vi "Peregrine_query_status.vi"(8 "error":errorcluster, 10 "Address":u8, 11 "Handle in":refnum<visa-resource-name>) -> (0 "error out":errorcluster, 1 "Speed":i16, 2 "Position":i32, 3 "Handle out":refnum<visa-resource-name>, 4 "Flags":T1)   [LabVIEW 2019]
panel:
  out "length":i32
  out "unsigned byte array":u8[](array[numeric])
  in  "Flags bundle":T1
  out "Command":i32
  out "Address":u8
  # "Inputs"
  # "Indicators"
  # "Outputs"
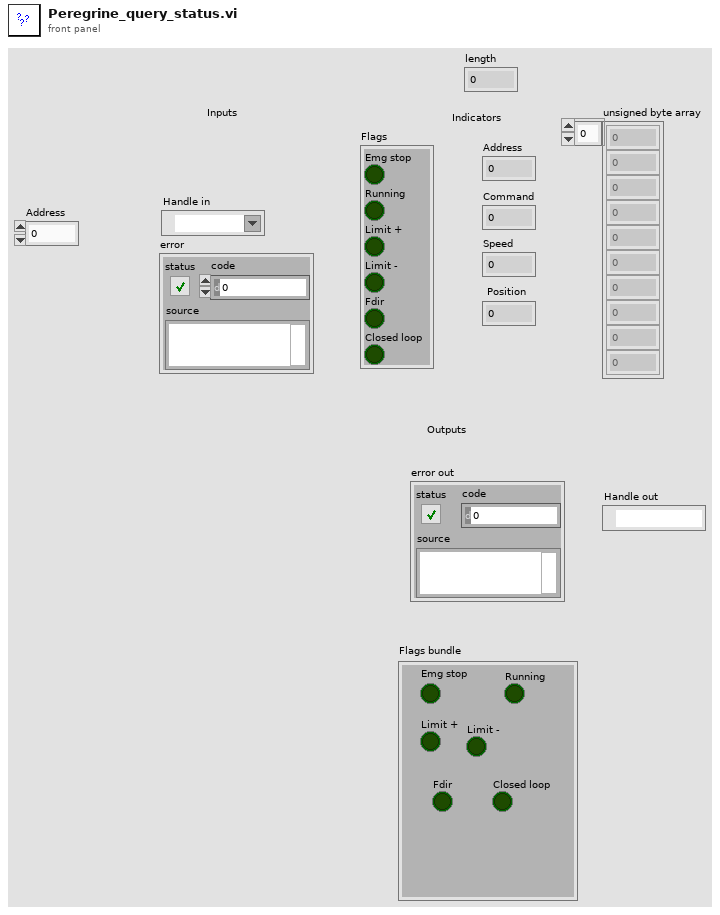
[diagram p1: front panel]
types:
  T1 = cluster{"Emg stop":bool, "Running":bool, "Limit +":bool, "Limit -":bool, "Fdir":bool, "Closed loop":bool}
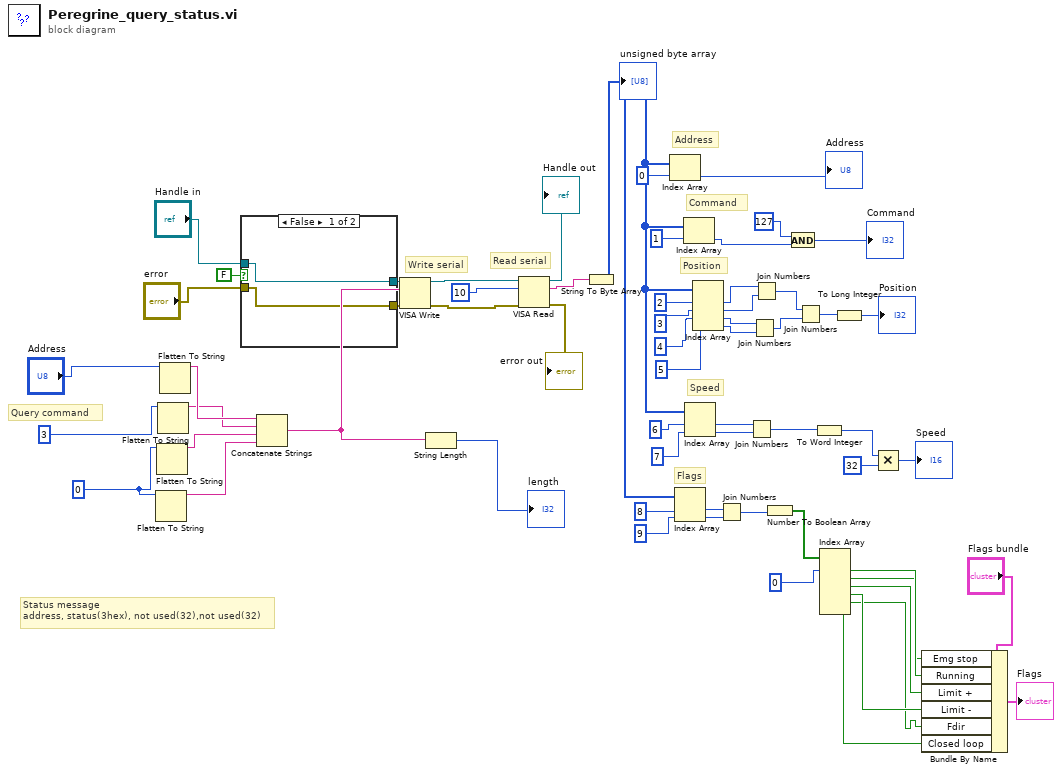
[diagram p0: block diagram]
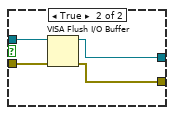
[diagram p2: hidden frame]
diagram:
  w6 = 0
  # "Write serial"
  # "Query command"
  # "Command"
  # "Address"
  # "Flags"
  # "Speed"
  # "Position"
  # "Read serial"
  # "Status message\naddress, status(3hex), not used(32),not used(32)"
  n1 = Flatten To String(anything=w6) -> (data string=w8:string)  [unwired: 3 in, 2 out]
  n2 = Flatten To String(anything=w6) -> (data string=w9:string)  [unwired: 3 in, 2 out]
  n3 = Flatten To String(anything=u8 3) -> (data string=w10:string)  [unwired: 3 in, 2 out]
  n4 = Flatten To String(anything="Address") -> (data string=w12:string)  [unwired: 3 in, 2 out]
  n5 = case shown="False" FALSE {
    tunnel: "Handle in" -> [w64 w68]
    tunnel: "error" -> [w63 w67]
    tunnel: [w63 w66] -> w3
    tunnel: [w64 w65] -> w2
    frame False {
    }
    frame True {
      n6 = VISA Flush I/O Buffer(VISA resource name=w68, error in (no error)=w67) -> (VISA resource name out=w65:refnum<visa-resource-name>, error out=w66:errorcluster)  [unwired: 1 in]
    }
  }
  n7 = Concatenate Strings(w12, w10, w9, w8) -> (w7:string)
  n8 = VISA Write(VISA resource name=w2, write buffer=w7, error in (no error)=w3) -> (VISA resource name out=w62:refnum<visa-resource-name>, error out=w26:errorcluster)  [unwired: 1 out]
  n9 = String Length(string=w7) -> (length=→"length":i32)
  n10 = VISA Read(VISA resource name=w62, byte count=10, error in (no error)=w26) -> (VISA resource name out=→"Handle out":refnum<visa-resource-name>, read buffer=w60:string, error out=→"error out":errorcluster)  [unwired: 1 out]
  n11 = String To Byte Array(string=w60) -> (unsigned byte array=w52:u8[])
  "unsigned byte array" <- w52
  n12 = Index Array(array=w52, index=0) -> (element=→"Address":u8)
  n13 = Index Array(array=w52, index #1=8, index #2=9) -> (element #1=w42:u8, element #2=w41:u8)
  n14 = Index Array(array=w52, index=1) -> (element=w44:u8)
  n15 = Index Array(array=w52, index #1=6, index #2=7) -> (element #1=w34:u8, element #2=w33:u8)
  n16 = Index Array(array=w52, index #1=2, index #2=3, index #3=4, index #4=5) -> (element #1=w50:u8, element #2=w49:u8, element #3=w48:u8, element #4=w47:u8)
  n17 = Join Numbers(hi=w42, lo=w41) -> ((hi.lo)=w39:u16)
  n18 = Join Numbers(hi=w34, lo=w33) -> ((hi.lo)=w32:u16)
  n19 = Join Numbers(hi=w48, lo=w47) -> ((hi.lo)=w46:u16)
  n20 = Join Numbers(hi=w50, lo=w49) -> ((hi.lo)=w45:u16)
  n21 = Number To Boolean Array(number=w39) -> (Boolean array=w37:bool[])
  n22 = And(x=127, y=w44) -> (x .and. y?=→"Command":i32)
  n23 = Join Numbers(hi=w45, lo=w46) -> ((hi.lo)=w40:u32)
  n24 = To Word Integer(number=w32) -> (16bit integer=w19:i16)
  n25 = Index Array(array=w37, index #1=0) -> (element #1=w16:bool, element #2=w15:bool, element #3=w24:bool, element #4=w23:bool, element #5=w22:bool, element #6=w21:bool)  [unwired: 5 in]
  n26 = To Long Integer(number=w40) -> (32bit integer=→"Position":i32)
  n27 = Multiply(x=w19, y=i16 32) -> (x*y=→"Speed":i16)
  n28 = Bundle By Name(cluster="Flags bundle", "Emg stop"=w15, "Running"=w16, "Limit +"=w24, "Limit -"=w23, "Fdir"=w22, "Closed loop"=w21) -> (→"Flags":T1)
